vi "ke37xx Trigger Overrun.vi"(0 "VISA Resource Name":refnum<visa-resource-name>, 5 "Trigger Type":T1(ring), 7 "Line (1)":u8=1, 11 "error in (no error)":errorcluster) -> (4 "VISA Resource Name Out":refnum<visa-resource-name>, 8 "Overrun":bool, 15 "error out":errorcluster)   [LabVIEW 2009, in "Keithley 3700 Series.lvlib"]
doc: "This VI allows you to query for an overrun condition on any of the trigger types available on the device.\n\nAn overrun condition occurs if an event was ignored because the event detector was already in the detected state when the event occurred."
uses:
  <instrlib>/Keithley 3706/Keithley 3700 Series.lvlib
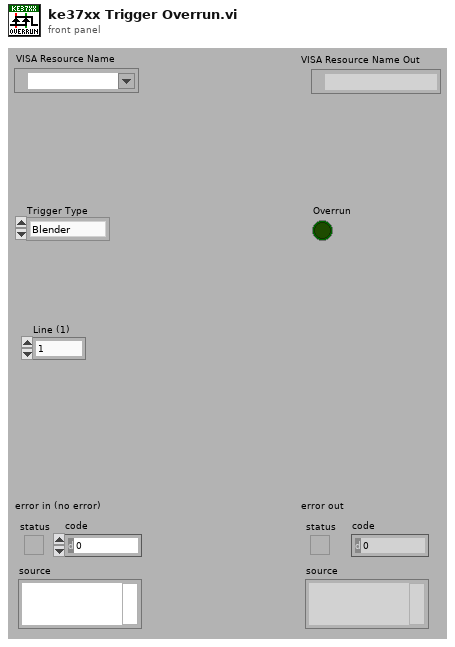
[diagram p1: front panel]
types:
  T1 = enum16{"Blender", "Digital I/O", "LAN", "TSP Link", "Timer"}
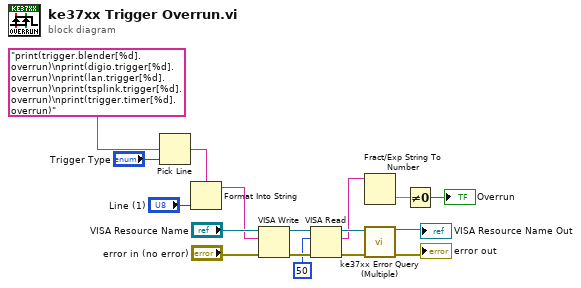
[diagram p0: block diagram]
diagram:
  n1 = Pick Line(multi-line string="print(trigger.blender[%d].overrun)\nprint(digio.trigger[%d].overrun)\nprint(lan.trigger[%d].overrun)\nprint(tsplink.trigger[%d].overrun)\nprint(trigger.timer[%d].overrun)", line index="Trigger Type") -> (output string=w3:string)  [unwired: 1 out]
  n2 = Format Into String(format string=w3, "Line (1)") -> (resulting string=w1:string)  [unwired: 2 in, 1 out]
  n3 = VISA Write(VISA resource name="VISA Resource Name", write buffer=w1, error in (no error)="error in (no error)") -> (VISA resource name out=w12:refnum<visa-resource-name>, error out=w13:errorcluster)  [unwired: 1 out]
  n4 = VISA Read(VISA resource name=w12, byte count=u32 50, error in (no error)=w13) -> (VISA resource name out=w11:refnum<visa-resource-name>, read buffer=w8:string, error out=w10:errorcluster)  [unwired: 1 out]
  n5 = Fract/Exp String To Number(string=w8) -> (number=w7:dbl)  [unwired: 4 out]
  n6 = call <instrlib>:"ke37xx Error Query (Multiple).vi"("VISA resource name"=w11, "error in (no error)"=w10) -> ("VISA resource name out"=→"VISA Resource Name Out":refnum<visa-resource-name>, "error out"=→"error out":errorcluster)  [unwired: 12 out]
  n7 = Not Equal To 0?(x=w7) -> (x != 0?=→"Overrun":bool)
